vi "Owner.vi"(7 "Action":T1, 8 "error in (no error)":errorcluster, 11 "Subpanel in":refnum<class "Subpanel.lvclass">) -> (0 "error out":errorcluster, 1 "Old Owner":refnum<class "Panel.lvclass">, 2 "I Was Owner?":bool)   [LabVIEW 2019, in "Panel.lvlib" / "Subpanel.lvclass"]
doc: "Gets/Sets the ownership status of the sub panel. Ownerships are used to determine if the current Panel is inserted in the panel or not.\n\n----\nPlease see the following web address for additional documentation and tutorial information:\nhttp://www.mooregoodideas.com/mgi-panel-manager/\n\nAuthor: Derek Trepanier\n\nCopyright (c) 2018, Moore Good Ideas, Inc.\n\nAll rights reserved.\n\nRedistribution and use in source and binary forms, with or without modification, are permitted provided that the following conditions are met:\n\n * Redistributions of source code must retain the above copyright notice, this list of conditions and the following disclaimer.\n * Redistributions in binary form must reproduce the above copyright notice, this list of conditions and the following disclaimer in the documentation and/or other materials provided with the distribution.\n * Neither the name of Moore Good Ideas, Inc. nor the names of its contributors may be used to endorse or promote products derived from this software without specific prior written permission.\n\nTHIS SOFTWARE IS PROVIDED BY THE COPYRIGHT HOLDERS AND CONTRIBUTORS \"AS IS\" AND ANY EXPRESS OR IMPLIED WARRANTIES, INCLUDING, BUT NOT LIMITED TO, THE IMPLIED WARRANTIES OF MERCHANTABILITY AND FITNESS FOR A PARTICULAR PURPOSE ARE DISCLAIMED. IN NO EVENT SHALL THE COPYRIGHT OWNER OR CONTRIBUTORS BE LIABLE FOR ANY DIRECT, INDIRECT, INCIDENTAL, SPECIAL, EXEMPLARY, OR CONSEQUENTIAL DAMAGES (INCLUDING, BUT NOT LIMITED TO, PROCUREMENT OF SUBSTITUTE GOODS OR SERVICES; LOSS OF USE, DATA, OR PROFITS; OR BUSINESS INTERRUPTION) HOWEVER CAUSED AND ON ANY THEORY OF LIABILITY, WHETHER IN CONTRACT, STRICT LIABILITY, OR TORT (INCLUDING NEGLIGENCE OR OTHERWISE) ARISING IN ANY WAY OUT OF THE USE OF THIS SOFTWARE, EVEN IF ADVISED OF THE POSSIBILITY OF SUCH DAMAGE."
uses:
  Subpanel.lvclass
  C:/Users/Public/Documents/Development/Drivers/Source/Utilities/Actor Framework Tools/Panel Manager/Panel/Panel/Panel.lvclass
  Action.ctl
  Panel.lvclass
  Subpanel.lvclass/Subpanel.ctl
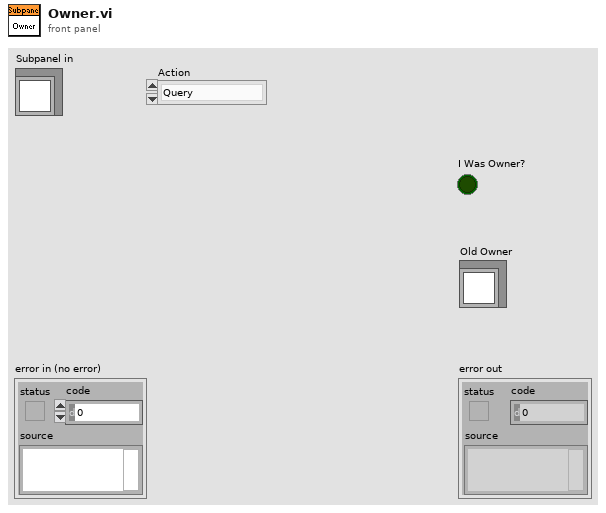
[diagram p1: front panel]
types:
  T1 = typedef "Panel.lvlib/Subpanel.lvclass/Action.ctl" = enum16{"Query", "Take", "Release"}
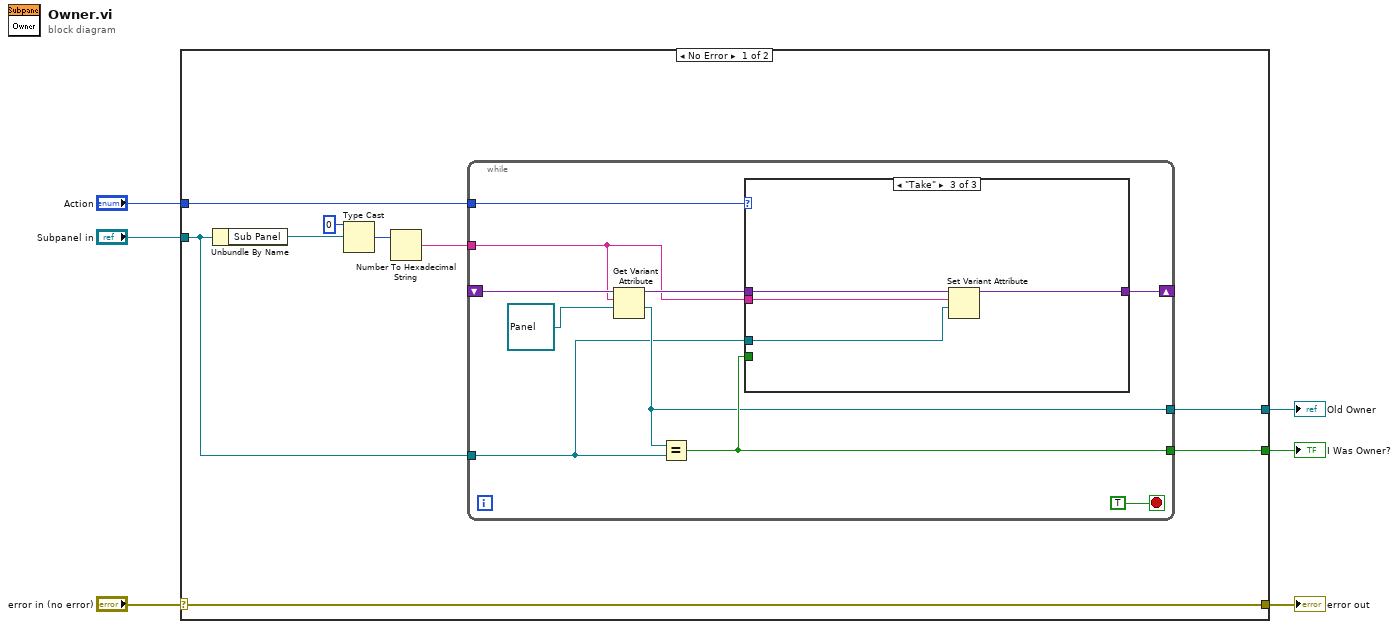
[diagram p0: block diagram]
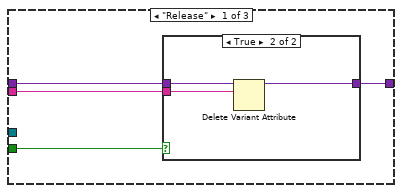
[diagram p2: hidden frame]
diagram:
  n1 = case shown="No Error" "error in (no error)" {
    selector: "error in (no error)" -> [w15 w39]
    tunnel: [w15 w39] -> w5
    tunnel: "Subpanel in" -> [w9 _]
    tunnel: "Action" -> [w14 _]
    tunnel: [w8 _] -> w2
    tunnel: [w7 _] -> w1
    frame No Error {
      n2 = Unbundle By Name(w9) -> ("Sub Panel"=w11:refnum<vi>)
      n3 = Type Cast(type=u32 0, x=w11) -> (*(type *) &x=w12:u32)
      n4 = Number To Hexadecimal String(2:w12) -> (0:w10:string)  [unwired: 1 in]
      n5 = while {
        tunnel: w10 -> [w21]
        shift-right: [w24] -> _
        shift-left: _ -> [w23]
        tunnel: w14 -> [w20]
        tunnel: w9 -> [w17]
        tunnel: [w19] -> w8
        tunnel: [w18] -> w7
        stop <- TRUE stop-if-true
        n6 = Get Variant Attribute(Variant=w23, name=w21, default value (empty Variant)=refnum<class "Panel.lvclass"> refnum ("Panel.lvlib:Panel.lvclass")) -> (duplicate Variant=w22:variant, value=w18:refnum<class "Panel.lvclass">)  [unwired: 1 in, 2 out]
        n7 = Equal?(x=w18, y=w17) -> (x = y?=w19:bool)
        n8 = case shown="\"Take\"" w20 {
          tunnel: [w28 w34 w38] -> w24
          tunnel: w22 -> [w29 w34 w37]
          tunnel: w21 -> [w27 _ w36]
          tunnel: w19 -> [w26 _ _]
          tunnel: w17 -> [_ _ w35]
          frame "Release" {
            n9 = case shown="True" w26 {
              tunnel: w29 -> [w30 w33]
              tunnel: [w30 w32] -> w28
              tunnel: w27 -> [_ w31]
              frame False {
                # "Someone else is the owner"
              }
              frame True {
                n10 = Delete Variant Attribute(6:w31, 7:w33) -> (3:w32:variant)  [unwired: 1 in, 2 out]
              }
            }
          }
          frame "Query" {
          }
          frame "Take" {
            n11 = Set Variant Attribute(Variant=w37, name=w36, value=w35) -> (Variant out=w38:variant)  [unwired: 1 in, 2 out]
          }
        }
      }
    }
    frame Error {
    }
  }
  "error out" <- w5
  "I Was Owner?" <- w2
  "Old Owner" <- w1
